vi "Expansion Board Analog Test.vi"() -> ()   [LabVIEW 2014]
uses:
  <vilib>/Rock Robotics/SystemInterfaces/AI/FPGA_AIChannel.ctl
  <vilib>/Rock Robotics/WPI/AnalogOutput/WPI_AnalogOutputChannel.ctl
panel:
  out "VIn RR 1":dbl
  out "VIn RR 0":dbl
  out "VIn RR 3":dbl
  out "VIn RR 2":dbl
  in  "Stop":bool
  out "Voltage In 3":dbl
  out "Voltage In 2":dbl
  out "Voltage In 1":dbl
  out "Voltage In 0":dbl
  in  "Voltage Out 1":dbl min=0.0 max=5.0
  in  "Voltage Out 0":dbl min=0.0 max=5.0
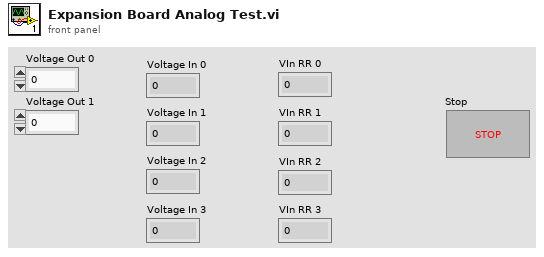
[diagram p1: front panel]
types:
  T1 = typedef "FPGA_AIChannel.ctl" = enum8{"AI 0", "AI 1", "AI 2", "AI 3", "AI MXP 0", "AI MXP 1", "AI MXP 2", "AI MXP 3", "Invalid"}
  T2 = typedef "WPI_AnalogOutputChannel.ctl" = enum8{"AO MXP 0", "AO MXP 1", "Invalid"}
  T3 = typedef "WPI_AnalogChannelDevRef.ctl" = cluster{"DevStatus":errorcluster, "Controller":T4, "Analog Channel":T1}
  T4 = typedef "FPGA_TypedefAnalogModule.ctl" = enum16{"Controller 1"}
  T5 = typedef "WPI_AOChannelDevRef.ctl" = cluster{"DevStatus":errorcluster, "Controller":T4, "AO Channel":T2}
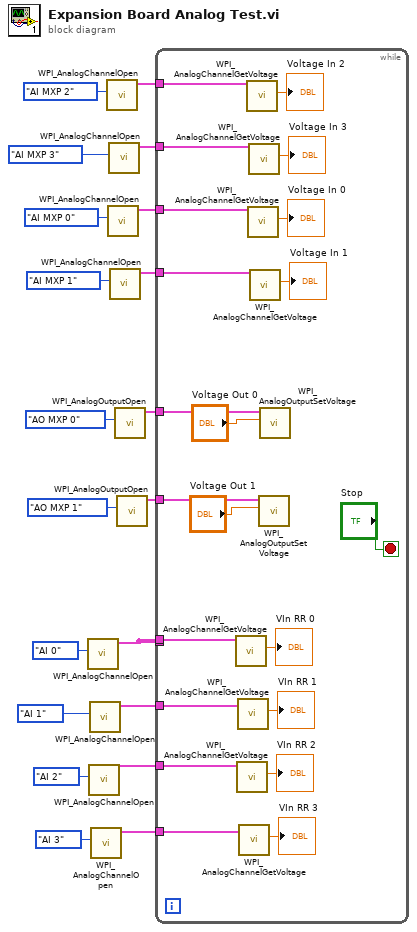
[diagram p0: block diagram]
diagram:
  n1 = call <vilib>:"WPI_AnalogChannelOpen.vi"("Analog Channel"=FPGA_AIChannel."AI 0") -> ("AIDeviceRef"=w4:T3)  [unwired: 9 in, 1 out]
  n2 = call <vilib>:"WPI_AnalogChannelOpen.vi"("Analog Channel"=FPGA_AIChannel."AI 2") -> ("AIDeviceRef"=w2:T3)  [unwired: 9 in, 1 out]
  n3 = call <vilib>:"WPI_AnalogChannelOpen.vi"("Analog Channel"=FPGA_AIChannel."AI 1") -> ("AIDeviceRef"=w3:T3)  [unwired: 9 in, 1 out]
  n4 = call <vilib>:"WPI_AnalogChannelOpen.vi"("Analog Channel"=FPGA_AIChannel."AI 3") -> ("AIDeviceRef"=w1:T3)  [unwired: 9 in, 1 out]
  n5 = call <vilib>:"WPI_AnalogChannelOpen.vi"("Analog Channel"=FPGA_AIChannel."AI MXP 2") -> ("AIDeviceRef"=w16:T3)  [unwired: 9 in, 1 out]
  n6 = call <vilib>:"WPI_AnalogChannelOpen.vi"("Analog Channel"=FPGA_AIChannel."AI MXP 0") -> ("AIDeviceRef"=w18:T3)  [unwired: 9 in, 1 out]
  n7 = call <vilib>:"WPI_AnalogChannelOpen.vi"("Analog Channel"=FPGA_AIChannel."AI MXP 3") -> ("AIDeviceRef"=w15:T3)  [unwired: 9 in, 1 out]
  n8 = call <vilib>:"WPI_AnalogChannelOpen.vi"("Analog Channel"=FPGA_AIChannel."AI MXP 1") -> ("AIDeviceRef"=w17:T3)  [unwired: 9 in, 1 out]
  n9 = call <vilib>:"WPI_AnalogOutputOpen.vi"("AO Channel"=WPI_AnalogOutputChannel."AO MXP 0") -> ("AODeviceRef"=w19:T5)  [unwired: 9 in, 1 out]
  n10 = call <vilib>:"WPI_AnalogOutputOpen.vi"("AO Channel"=WPI_AnalogOutputChannel."AO MXP 1") -> ("AODeviceRef"=w20:T5)  [unwired: 9 in, 1 out]
  n11 = while {
    tunnel: w20 -> [w41]
    tunnel: w19 -> [w40]
    tunnel: w18 -> [w37]
    tunnel: w17 -> [w35]
    tunnel: w16 -> [w33]
    tunnel: w15 -> [w31]
    tunnel: w4 -> [_]
    tunnel: w4 -> [w24]
    tunnel: w3 -> [w23]
    tunnel: w2 -> [w22]
    tunnel: w1 -> [w21]
    stop <- "Stop" stop-if-true
    n12 = call <vilib>:"WPI_AnalogChannelGetVoltage.vi"("AIDeviceRef"=w24) -> ("Voltage"=→"VIn RR 0":dbl)  [unwired: 8 in, 2 out]
    n13 = call <vilib>:"WPI_AnalogChannelGetVoltage.vi"("AIDeviceRef"=w22) -> ("Voltage"=→"VIn RR 2":dbl)  [unwired: 8 in, 2 out]
    n14 = call <vilib>:"WPI_AnalogChannelGetVoltage.vi"("AIDeviceRef"=w23) -> ("Voltage"=→"VIn RR 1":dbl)  [unwired: 8 in, 2 out]
    n15 = call <vilib>:"WPI_AnalogChannelGetVoltage.vi"("AIDeviceRef"=w21) -> ("Voltage"=→"VIn RR 3":dbl)  [unwired: 8 in, 2 out]
    n16 = call <vilib>:"WPI_AnalogChannelGetVoltage.vi"("AIDeviceRef"=w33) -> ("Voltage"=→"Voltage In 2":dbl)  [unwired: 8 in, 2 out]
    n17 = call <vilib>:"WPI_AnalogChannelGetVoltage.vi"("AIDeviceRef"=w37) -> ("Voltage"=→"Voltage In 0":dbl)  [unwired: 8 in, 2 out]
    n18 = call <vilib>:"WPI_AnalogChannelGetVoltage.vi"("AIDeviceRef"=w31) -> ("Voltage"=→"Voltage In 3":dbl)  [unwired: 8 in, 2 out]
    n19 = call <vilib>:"WPI_AnalogChannelGetVoltage.vi"("AIDeviceRef"=w35) -> ("Voltage"=→"Voltage In 1":dbl)  [unwired: 8 in, 2 out]
    n20 = call <vilib>:"WPI_AnalogOutputSetVoltage.vi"("Voltage"="Voltage Out 1", "AODeviceRef"=w41) -> ()  [unwired: 8 in, 2 out]
    n21 = call <vilib>:"WPI_AnalogOutputSetVoltage.vi"("Voltage"="Voltage Out 0", "AODeviceRef"=w40) -> ()  [unwired: 8 in, 2 out]
  }
